vi "Read Strings.vi"(8 "error in (no error)":errorcluster, 11 "Ring D Element in":refnum<class "String dropdown D Element.lvclass">) -> (0 "error out":errorcluster, 2 "Strings":string[](array[string]), 3 "Ring D Element out":refnum<class "String dropdown D Element.lvclass">)   [LabVIEW 2018, in "D Datagrid Library.lvlib" / "String dropdown D Element.lvclass"]
uses:
  String dropdown D Element.lvclass
  String dropdown D Element.lvclass/String dropdown D Element.ctl
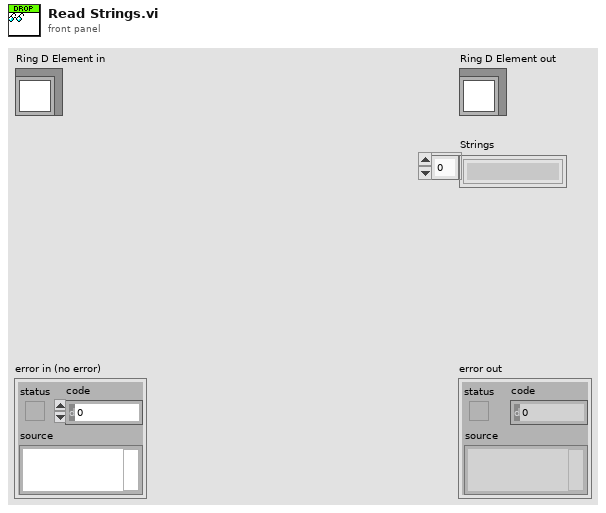
[diagram p1: front panel]
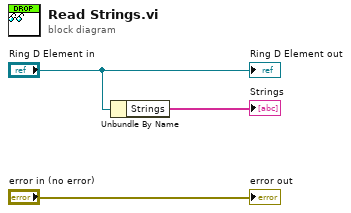
[diagram p0: block diagram]
diagram:
  n1 = Unbundle By Name("Ring D Element in") -> ("Strings"=→"Strings":string[])
  "error out" <- "error in (no error)"
  "Ring D Element out" <- "Ring D Element in"
